vi "Apply Offset Angle.vi"(7 "save to file (F)":bool, 8 "error in (no error)":errorcluster, 10 "ccw offset angle (rad)":dbl, 11 "servo motor in":refnum<class "NI_Robotics_Starter Kit Servo Motor.lvclass">) -> (0 "error out":errorcluster, 3 "servo motor out":refnum<class "NI_Robotics_Starter Kit Servo Motor.lvclass">)   [LabVIEW 2017, in "NI_Robotics_Starter Kit Servo Motor.lvclass"]
uses:
  <vilib>/robotics/Starter Kit/Servo Motor/NI_Robotics_Starter Kit Servo Motor.lvclass
  <vilib>/robotics/Starter Kit/Servo Motor/NI_Robotics_Starter Kit Servo Motor.lvclass/NI_Robotics_Starter Kit Servo Motor.ctl
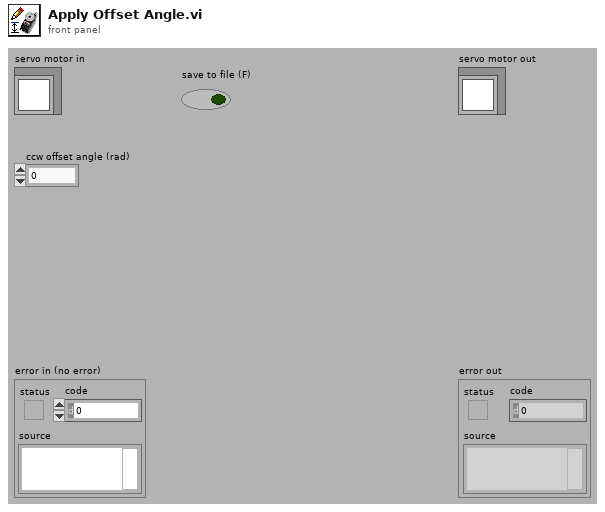
[diagram p1: front panel]
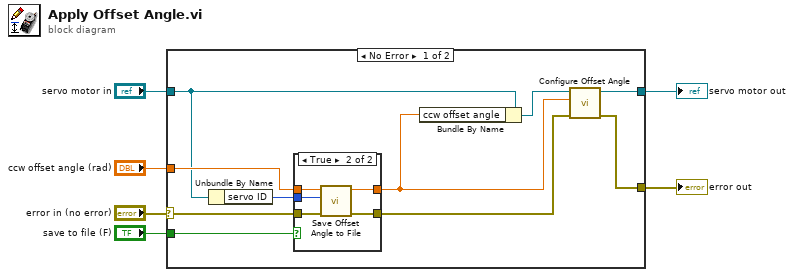
[diagram p0: block diagram]
diagram:
  n1 = case shown="No Error" "error in (no error)" {
    selector: "error in (no error)" -> [w15 w25]
    tunnel: [w12 w25] -> w5
    tunnel: "servo motor in" -> [w8 w24]
    tunnel: [w13 w24] -> w3
    tunnel: "save to file (F)" -> [w16 _]
    tunnel: "ccw offset angle (rad)" -> [w10 _]
    frame No Error {
      n2 = Unbundle By Name(w8) -> ("servo ID"=w14:i32)
      n3 = case shown="True" w16 {
        tunnel: w15 -> [w18 w23]
        tunnel: w14 -> [_ w22]
        tunnel: w10 -> [w17 w21]
        tunnel: [w18 w20] -> w11
        tunnel: [w17 w19] -> w9
        frame False {
        }
        frame True {
          n4 = call <vilib>:"Save Offset Angle to File.vi"("error in (no error)"=w23, "servo ID (0)"=w22, "ccw offset angle (rad)"=w21) -> ("error out"=w20:errorcluster, "coerced ccw offset angle (rad)"=w19:dbl)  [unwired: 6 in, 1 out]
        }
      }
      n5 = Bundle By Name(cluster=w8, "ccw offset angle"=w9) -> (w7:refnum<class "NI_Robotics_Starter Kit Servo Motor.lvclass">)
      n6 = call-dynamic "Configure Offset Angle.vi"("error in (no error)"=w11, "ccw offset angle (rad)"=w9, "NI_Robotics_Starter Kit Servo Motor in"=w7) -> ("error out"=w12:errorcluster, "NI_Robotics_Starter Kit Servo Motor out"=w13:refnum<class "NI_Robotics_Starter Kit Servo Motor.lvclass">)  [unwired: 7 in]
    }
    frame Error {
    }
  }
  "error out" <- w5
  "servo motor out" <- w3
